vi "Get associated LV error.vi"(11 "IAbortOrErrorHandler in":refnum<class "IAbortOrErrorHandler.lvclass">) -> (2 "Associated LabVIEW Error":errorcluster, 3 "IAbortOrErrorHandler out":refnum<class "IAbortOrErrorHandler.lvclass">)   [LabVIEW 2020, in "wamplv.lvlib" / "IAbortOrErrorHandler.lvclass"]
uses:
  Error/IAbortOrErroHandler/IAbortOrErrorHandler.lvclass
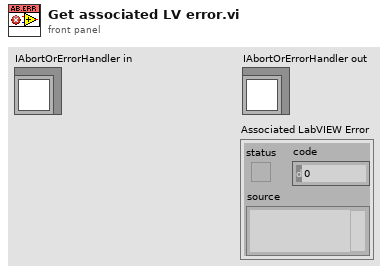
[diagram p1: front panel]
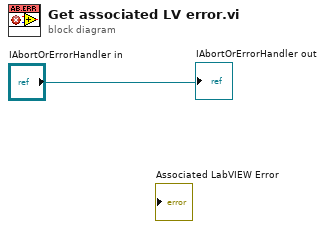
[diagram p0: block diagram]
diagram:
  "IAbortOrErrorHandler out" <- "IAbortOrErrorHandler in"
